vi "IPC-Modbus-Transfer.vi"(0 "connection ID in":refnum<k5>, 2 "CmdQRef":refnum<queue>, 5 "VISA resource name":refnum<visa-resource-name>="COM2" caption="VISA资源名称", 7 "baud rate (9600)":u32=9600 caption="波特率(9600)", 9 "parity (Even)":u16(ring)=2 caption="奇偶（偶）" items=["无", "奇", "偶"], 11 "错误输入（无错误）":errorcluster) -> (4 "connection ID out":refnum<k5>, 15 "错误输出":errorcluster)   [LabVIEW 2014]
panel:
  out "*(类型 *) &x":u8[](array[numeric])
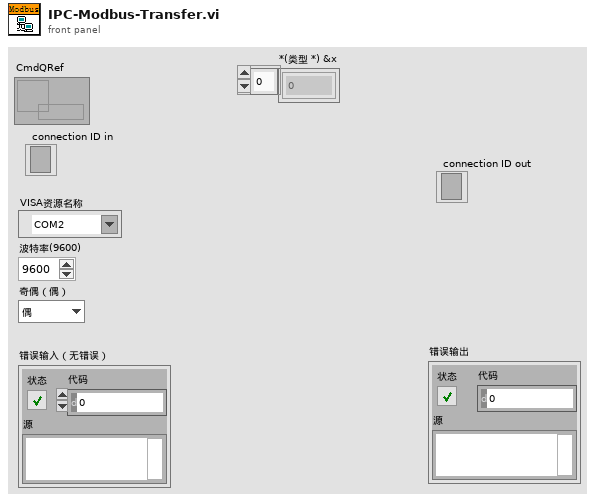
[diagram p1: front panel]
types:
  T1 = cluster{"Transaction ID":u16, "Protocol ID":u16, "Length":u16, " Unit ID":u8}
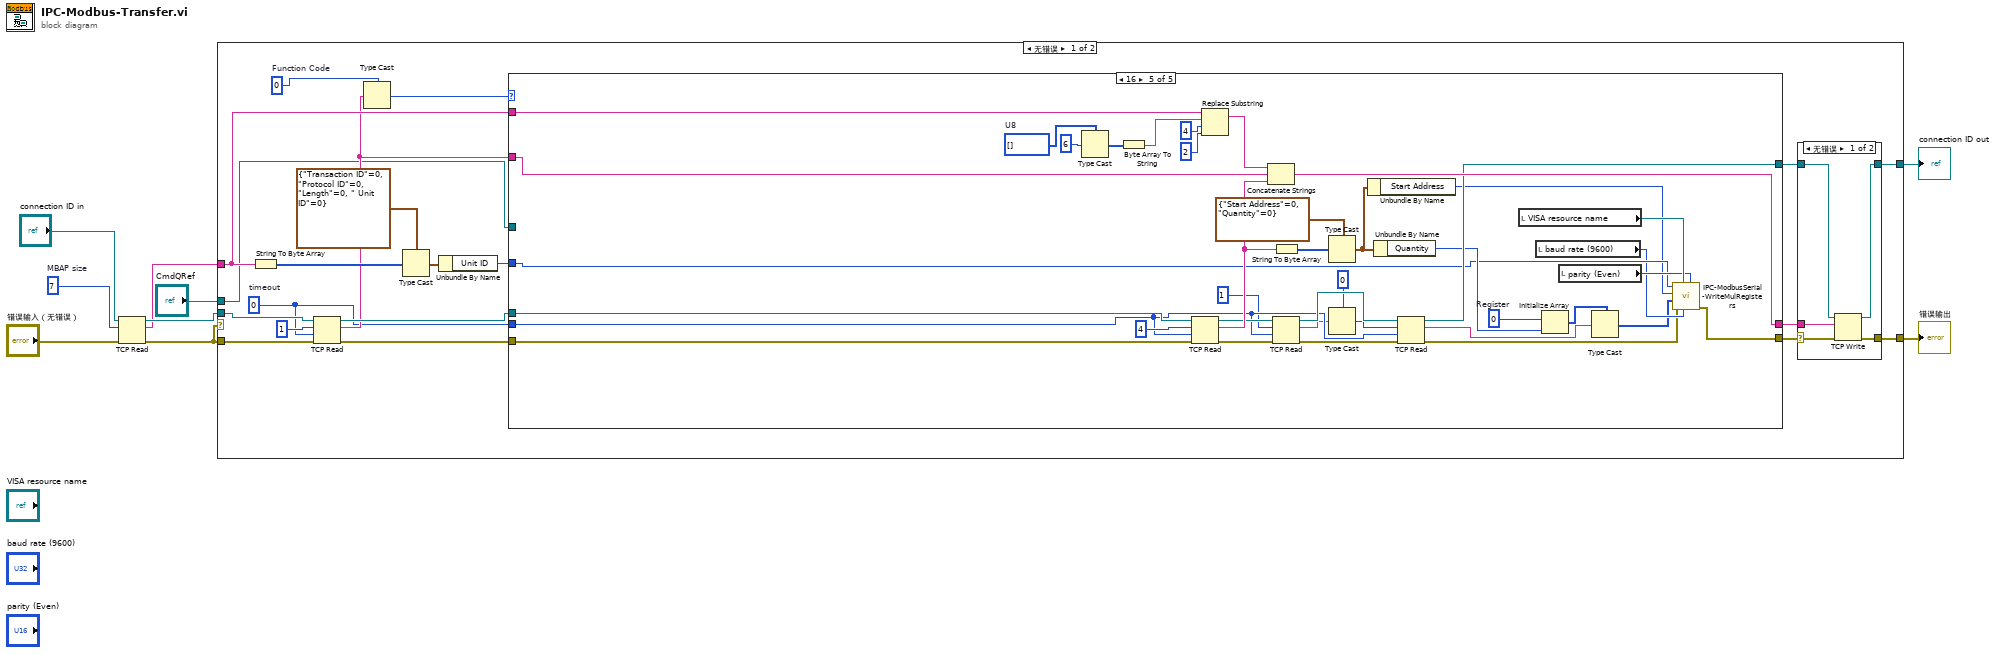
[diagram p0: block diagram]
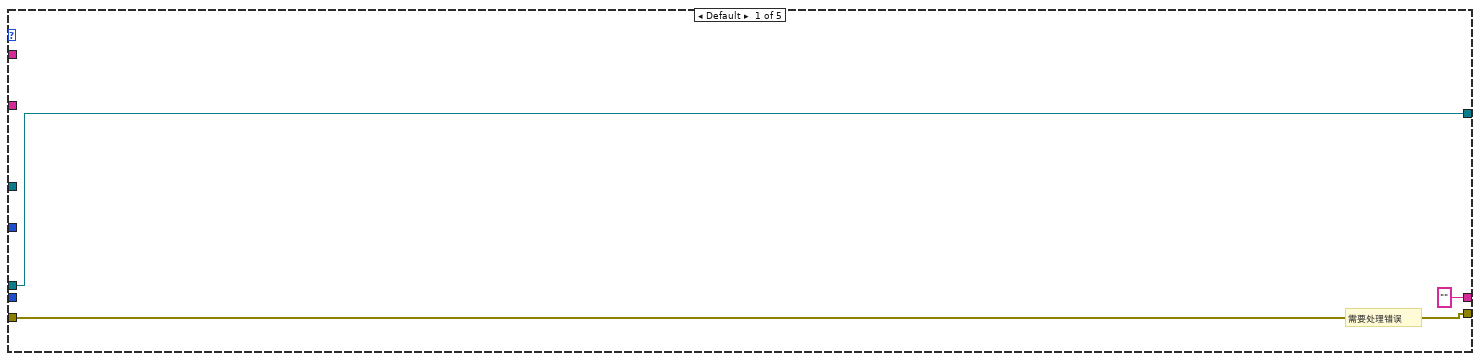
[diagram p2: hidden frame]
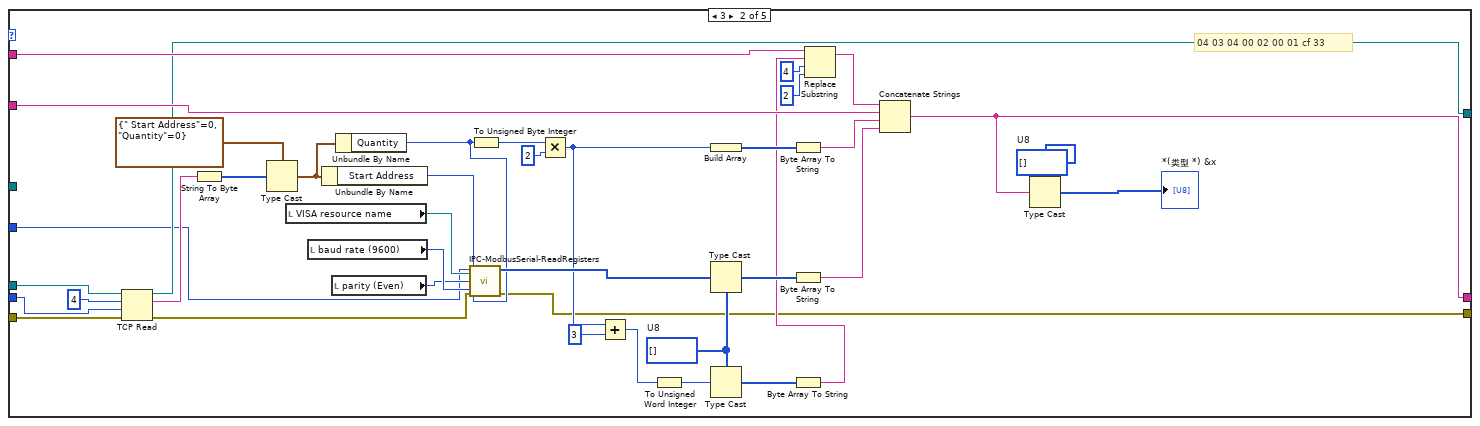
[diagram p3: hidden frame]
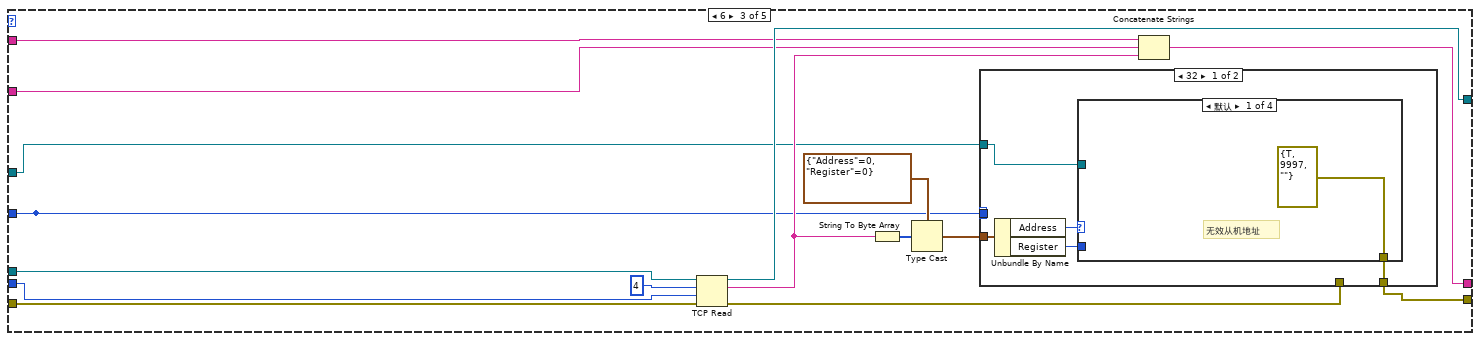
[diagram p4: hidden frame]
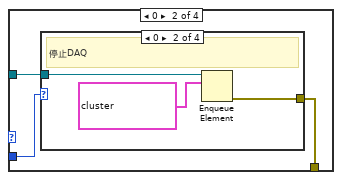
[diagram p5: hidden frame]
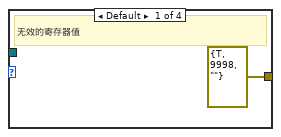
[diagram p6: hidden frame]
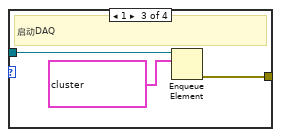
[diagram p7: hidden frame]
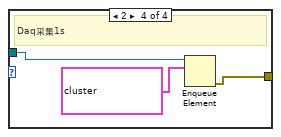
[diagram p8: hidden frame]
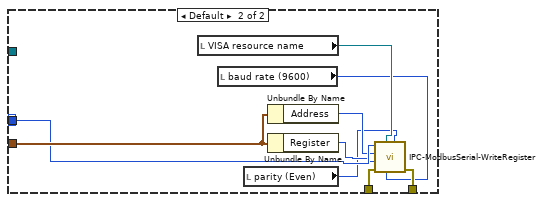
[diagram p11: hidden frame]
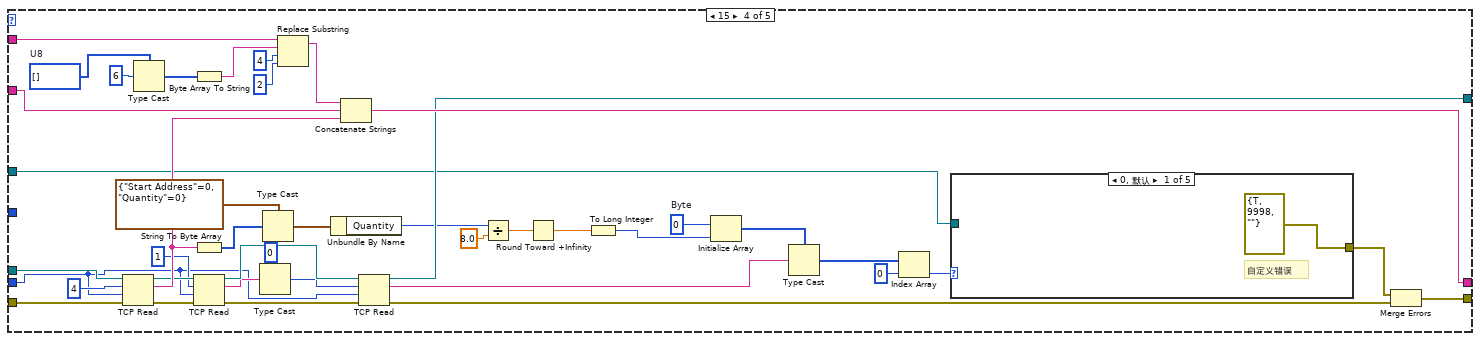
[diagram p12: hidden frame]
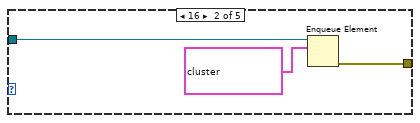
[diagram p13: hidden frame]
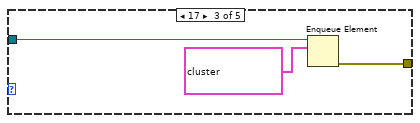
[diagram p14: hidden frame]
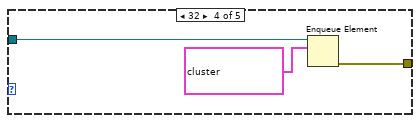
[diagram p15: hidden frame]
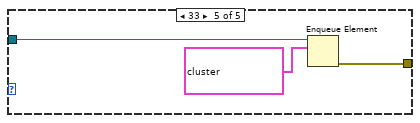
[diagram p16: hidden frame]
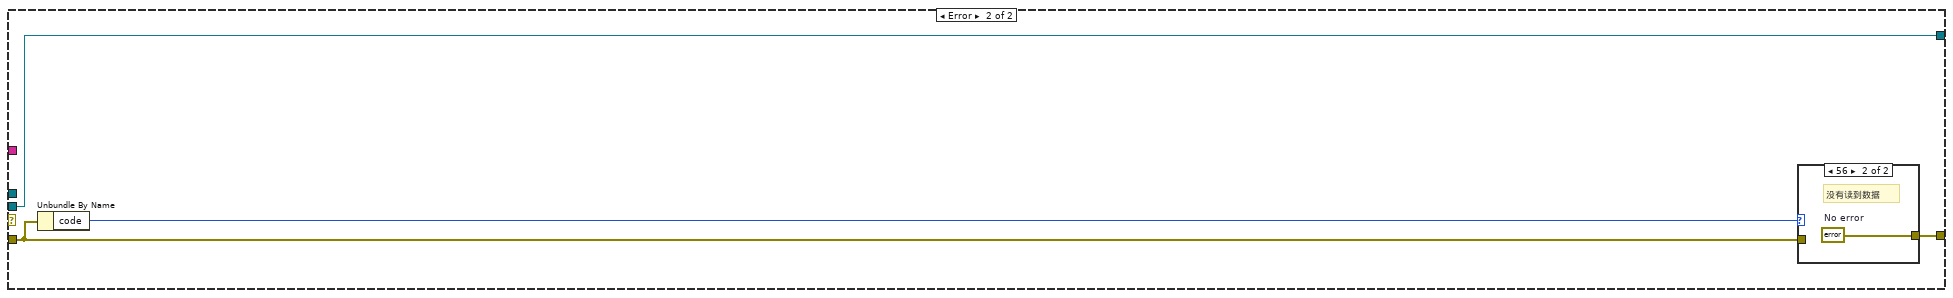
[diagram p18: hidden frame]
diagram:
  w9 = 7  # MBAP size
  n1 = TCP Read(connection ID="connection ID in", bytes to read=w9, error in (no error)="错误输入（无错误）") -> (connection ID out=w8:refnum<k5>, data out=w7:string, error out=w6:errorcluster)  [unwired: 2 out]
  n2 = case shown="无错误" w6 {
    tunnel: w8 -> [w29 w220]
    tunnel: [w28 w220] -> w4
    tunnel: [w27 w218] -> w5
    tunnel: w7 -> [w26 _]
    tunnel: w6 -> [w16 w217]
    tunnel: "CmdQRef" -> [w10 _]
    frame No Error {
      w14 = 0  # timeout
      w21 = u8 0  # Function Code
      n3 = String To Byte Array(string=w26) -> (unsigned byte array=w25:u8[])
      n4 = TCP Read(connection ID=w29, bytes to read=1 ("读取的字节"), error in (no error)=w16, 9:w14) -> (connection ID out=w24:refnum<k5>, data out=w19:string, error out=w23:errorcluster)  [unwired: 1 out]
      n5 = Type Cast(type=w21, x=w19) -> (*(type *) &x=w11:u8)
      n6 = Type Cast(type=T1 {"Transaction ID"=0, "Protocol ID"=0, "Length"=0, " Unit ID"=0}, x=w25) -> (*(type *) &x=w13:T1)
      n7 = Unbundle By Name(w13) -> ("Unit ID"=w17:u8)
      n8 = case shown="16" w11 {
        tunnel: w26 -> [_ w49 w81 w118 w187]
        tunnel: w24 -> [w32 w46 w84 w142 w209]
        tunnel: w23 -> [w31 w45 w83 w141 w208]
        tunnel: w19 -> [_ w48 w80 w140 w205]
        tunnel: ["" w38 w79 w143 w203] -> w18
        tunnel: w17 -> [_ w40 w75 _ w176]
        tunnel: [w32 w44 w85 w139 w198] -> w15
        tunnel: w14 -> [_ w47 w82 w130 w196]
        tunnel: [w31 w34 w73 w127 w171] -> w12
        tunnel: w10 -> [_ _ w74 w128 _]
        frame Default {
          # "需要处理错误"
        }
        frame 3 {
          w37 = u8[] []  # U8
          w54 = u8[] []  # U8
          # "04 03 04 00 02 00 01 cf 33"
          n9 = TCP Read(connection ID=w46, bytes to read=4 ("读取的字节"), error in (no error)=w45, 9:w47) -> (connection ID out=w44:refnum<k5>, data out=w69:string, error out=w33:errorcluster)  [unwired: 1 out]
          n10 = String To Byte Array(string=w69) -> (unsigned byte array=w70:u8[])
          n11 = Type Cast(type=cluster{" Start Address":u16, "Quantity":u16} {" Start Address"=0, "Quantity"=0}, x=w70) -> (*(type *) &x=w66:cluster{" Start Address":u16, "Quantity":u16})
          n12 = local read "VISA resource name"() -> (w42:refnum<visa-resource-name>)
          n13 = local read "baud rate (9600)"() -> (w43:u32)
          n14 = Unbundle By Name(w66) -> ("Start Address"=w68:u16)
          n15 = local read "parity (Even)"() -> (w41:u16)
          n16 = Unbundle By Name(w66) -> ("Quantity"=w61:u16)
          n17 = call "IPC-ModbusSerial-ReadRegisters.vi"("parity (Even)"=w41, "baud rate (9600)"=w43, "VISA resource name"=w42, "error in (no error)"=w33, "number of holding registers"=w61, "starting address"=w68, "unit ID"=w40) -> ("error out"=w34:errorcluster, "register values"=w62:u16[])  [unwired: 2 in]
          n18 = To Unsigned Byte Integer(number=w61) -> (unsigned 8bit integer=w60:u8)
          n19 = Multiply(x=w60, y=u8 2) -> (x*y=w52:u8)
          n20 = Add(x=w52, y=3) -> (x+y=w53:i32)
          n21 = To Unsigned Word Integer(number=w53) -> (unsigned 16bit integer=w51:u16)
          n22 = Build Array(w52) -> (w64:u8[])
          n23 = Type Cast(type=w54, x=w62) -> (*(type *) &x=w59:u8[])
          n24 = Type Cast(type=w54, x=w51) -> (*(type *) &x=w55:u8[])
          n25 = Byte Array To String(unsigned byte array=w64) -> (string=w58:string)
          n26 = Byte Array To String(unsigned byte array=w59) -> (string=w63:string)
          n27 = Byte Array To String(unsigned byte array=w55) -> (string=w35:string)
          n28 = Replace Substring(2:2 ("长度（子字符串长度）"), 3:4 ("偏移量(0)"), 4:w35, 5:w49) -> (1:w50:string)  [unwired: 1 out]
          n29 = Concatenate Strings(w50, w48, w58, w63) -> (w38:string)
          n30 = Type Cast(type=w37, x=w38) -> (*(type *) &x=→"*(类型 *) &x":u8[])
        }
        frame 6 {
          n31 = TCP Read(connection ID=w84, bytes to read=4 ("读取的字节"), error in (no error)=w83, 9:w82) -> (connection ID out=w85:refnum<k5>, data out=w86:string, error out=w72:errorcluster)  [unwired: 1 out]
          n32 = String To Byte Array(string=w86) -> (unsigned byte array=w78:u8[])
          n33 = Type Cast(type=cluster{"Address":u16, "Register":u16} {"Address"=0, "Register"=0}, x=w78) -> (*(type *) &x=w76:cluster{"Address":u16, "Register":u16})
          n34 = case shown="32" w75 {
            selector: w75 -> [_ w113]
            tunnel: [w88 w115] -> w73
            tunnel: w75 -> [_ _]
            tunnel: w76 -> [w92 w114]
            tunnel: w74 -> [w89 _]
            tunnel: w72 -> [_ w107]
            frame 32 {
              n35 = Unbundle By Name(w92) -> ("Address"=w91:u16, "Register"=w90:u16)
              n36 = case shown="默认" w91 {
                tunnel: w90 -> [_ w96 _ _]
                tunnel: w89 -> [_ w95 _ _]
                tunnel: [errorcluster {"status"=TRUE, "code"=9997, "source"=""} ("错误常量") w94 _ _] -> w88
                frame Default {
                  # "无效从机地址"
                }
                frame 0 {
                  n37 = case shown="0" w96 {
                    tunnel: w95 -> [_ w99 w101 w104]
                    tunnel: [errorcluster {"status"=TRUE, "code"=9998, "source"=""} ("错误常量") w98 w102 w105] -> w94
                    frame Default {
                      # "无效的寄存器值"
                    }
                    frame 0 {
                      # "停止DAQ"
                      n38 = Enqueue Element(queue=w99, element=cluster{"Data":variant, "State":string} {"Data"=variant, "State"="Cmd::StopDaq"} ("元素")) -> (error out=w98:errorcluster)  [unwired: 2 in, 2 out]
                    }
                    frame 1 {
                      # "启动DAQ"
                      n39 = Enqueue Element(queue=w101, element=cluster{"Data":variant, "State":string} {"Data"=variant, "State"="Cmd::StartDaq"} ("元素")) -> (error out=w102:errorcluster)  [unwired: 2 in, 2 out]
                    }
                    frame 2 {
                      # "Daq采集1s"
                      n40 = Enqueue Element(queue=w104, element=cluster{"Data":variant, "State":string} {"Data"=variant, "State"="Cmd::DaqOnce"} ("元素")) -> (error out=w105:errorcluster)  [unwired: 2 in, 2 out]
                    }
                  }
                }
                frame 1 {
                  # "设置6133频率"
                }
                frame 2 {
                  # "设置6220频率"
                }
              }
            }
            frame Default {
              n41 = local read "VISA resource name"() -> (w112:refnum<visa-resource-name>)
              n42 = local read "baud rate (9600)"() -> (w109:u32)
              n43 = local read "parity (Even)"() -> (w108:u16)
              n44 = Unbundle By Name(w114) -> ("Address"=w111:u16)
              n45 = Unbundle By Name(w114) -> ("Register"=w110:u16)
              n46 = call "IPC-ModbusSerial-WriteRegister.vi"("parity (Even)"=w108, "baud rate (9600)"=w109, "VISA resource name"=w112, "error in (no error)"=w107, "holding register value"=w110, "address"=w111, "unit ID"=w113) -> ("error out"=w115:errorcluster)  [unwired: 4 in]
            }
          }
          n47 = Concatenate Strings(w81, w80, w86) -> (w79:string)
        }
        frame 15 {
          w120 = u8[] []  # U8
          w147 = u8 0  # Byte
          n48 = TCP Read(connection ID=w142, bytes to read=4 ("读取的字节"), error in (no error)=w141, 9:w130) -> (connection ID out=w153:refnum<k5>, data out=w155:string, error out=w152:errorcluster)  [unwired: 1 out]
          n49 = Type Cast(type=w120, x=u16 6) -> (*(type *) &x=w122:u8[])
          n50 = Byte Array To String(unsigned byte array=w122) -> (string=w119:string)
          n51 = String To Byte Array(string=w155) -> (unsigned byte array=w156:u8[])
          n52 = TCP Read(connection ID=w153, bytes to read=1 ("读取的字节"), error in (no error)=w152, 9:w130) -> (connection ID out=w151:refnum<k5>, data out=w149:string, error out=w150:errorcluster)  [unwired: 1 out]
          n53 = Type Cast(type=u8 0, x=w149) -> (*(type *) &x=w135:u8)
          n54 = Type Cast(type=cluster{"Start Address":u16, "Quantity":u16} {"Start Address"=0, "Quantity"=0}, x=w156) -> (*(type *) &x=w144:cluster{"Start Address":u16, "Quantity":u16})
          n55 = Replace Substring(2:2 ("长度（子字符串长度）"), 3:4 ("偏移量(0)"), 4:w119, 5:w118) -> (1:w117:string)  [unwired: 1 out]
          n56 = Unbundle By Name(w144) -> ("Quantity"=w134:u16)
          n57 = Concatenate Strings(w117, w140, w155) -> (w143:string)
          n58 = TCP Read(connection ID=w151, bytes to read=w135, error in (no error)=w150, 9:w130) -> (connection ID out=w139:refnum<k5>, data out=w145:string, error out=w126:errorcluster)  [unwired: 1 out]
          n59 = Divide(x=w134, y=8.0) -> (x/y=w138:dbl)
          n60 = Round Toward +Infinity(x=w138) -> (ceil(x): smallest int >= x=w137:dbl)
          n61 = To Long Integer(number=w137) -> (32bit integer=w133:i32)
          n62 = Initialize Array(w147, w133) -> (w146:u8[])
          n63 = Type Cast(type=w146, x=w145) -> (*(type *) &x=w132:u8[])
          n64 = Index Array(array=w132, index=0 ("索引")) -> (element=w129:u8)
          n65 = case shown="0, 默认" w129 {
            tunnel: w128 -> [_ w161 w163 w166 w169]
            tunnel: [errorcluster {"status"=TRUE, "code"=9998, "source"=""} ("错误常量") w160 w162 w165 w168] -> w125
            frame 0, Default {
              # "自定义错误"
            }
            frame 16 {
              n66 = Enqueue Element(queue=w161, element=cluster{"Data":variant, "State":string} {"Data"=variant, "State"="Cmd::StartDaq"} ("元素")) -> (error out=w160:errorcluster)  [unwired: 2 in, 2 out]
            }
            frame 17 {
              n67 = Enqueue Element(queue=w163, element=cluster{"Data":variant, "State":string} {"Data"=variant, "State"="Cmd::StopDaq"} ("元素")) -> (error out=w162:errorcluster)  [unwired: 2 in, 2 out]
            }
            frame 32 {
              n68 = Enqueue Element(queue=w166, element=cluster{"Data":variant, "State":string} {"Data"=variant, "State"="Cmd::StartUdp"} ("元素")) -> (error out=w165:errorcluster)  [unwired: 2 in, 2 out]
            }
            frame 33 {
              n69 = Enqueue Element(queue=w169, element=cluster{"Data":variant, "State":string} {"Data"=variant, "State"="Cmd::StopUdp"} ("元素")) -> (error out=w168:errorcluster)  [unwired: 2 in, 2 out]
            }
          }
          n70 = Merge Errors(w125, w126) -> (w127:errorcluster)
        }
        frame 16 {
          w181 = u8[] []  # U8
          w192 = u16 0  # Register
          n71 = Type Cast(type=w181, x=u16 6) -> (*(type *) &x=w183:u8[])
          n72 = Byte Array To String(unsigned byte array=w183) -> (string=w180:string)
          n73 = TCP Read(connection ID=w209, bytes to read=4 ("读取的字节"), error in (no error)=w208, 9:w196) -> (connection ID out=w201:refnum<k5>, data out=w204:string, error out=w200:errorcluster)  [unwired: 1 out]
          n74 = Replace Substring(2:2 ("长度（子字符串长度）"), 3:4 ("偏移量(0)"), 4:w180, 5:w187) -> (1:w186:string)  [unwired: 1 out]
          n75 = Concatenate Strings(w186, w205, w204) -> (w203:string)
          n76 = String To Byte Array(string=w204) -> (unsigned byte array=w206:u8[])
          n77 = TCP Read(connection ID=w201, bytes to read=1 ("读取的字节"), error in (no error)=w200, 9:w196) -> (connection ID out=w199:refnum<k5>, data out=w195:string, error out=w197:errorcluster)  [unwired: 1 out]
          n78 = Type Cast(type=cluster{"Start Address":u16, "Quantity":u16} {"Start Address"=0, "Quantity"=0}, x=w206) -> (*(type *) &x=w188:cluster{"Start Address":u16, "Quantity":u16})
          n79 = Type Cast(type=u8 0, x=w195) -> (*(type *) &x=w194:u8)
          n80 = Unbundle By Name(w188) -> ("Start Address"=w175:u16)
          n81 = Unbundle By Name(w188) -> ("Quantity"=w191:u16)
          n82 = TCP Read(connection ID=w199, bytes to read=w194, error in (no error)=w197, 9:w196) -> (connection ID out=w198:refnum<k5>, data out=w189:string, error out=w172:errorcluster)  [unwired: 1 in]
          n83 = local read "VISA resource name"() -> (w178:refnum<visa-resource-name>)
          n84 = local read "baud rate (9600)"() -> (w174:u32)
          n85 = Initialize Array(w192, w191) -> (w190:u16[])
          n86 = local read "parity (Even)"() -> (w177:u16)
          n87 = Type Cast(type=w190, x=w189) -> (*(type *) &x=w173:u16[])
          n88 = call "IPC-ModbusSerial-WriteMulRegisters.vi"("parity (Even)"=w177, "baud rate (9600)"=w174, "VISA resource name"=w178, "error in (no error)"=w172, "holding register values"=w173, "starting address"=w175, "unit ID"=w176) -> ("error out"=w171:errorcluster)  [unwired: 4 in]
        }
      }
      n89 = case shown="无错误" w12 {
        selector: w12 -> [w213 w215]
        tunnel: [w212 w215] -> w27
        tunnel: [w210 w216] -> w28
        tunnel: w15 -> [w211 w216]
        tunnel: w18 -> [w214 _]
        frame No Error {
          n90 = TCP Write(connection ID=w211, data in=w214, error in (no error)=w213) -> (connection ID out=w210:refnum<k5>, error out=w212:errorcluster)  [unwired: 1 in, 1 out]
        }
        frame Error {
        }
      }
    }
    frame Error {
      n91 = Unbundle By Name(w217) -> ("code"=w219:i32)
      n92 = case shown="56" w219 {
        tunnel: [w221 w222] -> w218
        tunnel: w217 -> [w221 _]
        frame Default {
        }
        frame 56 {
          w222 = errorcluster {"status"=FALSE, "code"=0, "source"=""}  # No error
          # "没有读到数据"
        }
      }
    }
  }
  "错误输出" <- w5
  "connection ID out" <- w4
